vi "Connect.vi"(8 "error in (no error)":errorcluster, 11 "Red Pitaya in":refnum<class "Red Pitaya.lvclass">) -> (0 "error out":errorcluster, 3 "Red Pitaya out":refnum<class "Red Pitaya.lvclass">)   [LabVIEW 2015]
uses:
  Mag Lab Measure/Mag Lab Error Handler/Mag Lab Error Handler.lvclass
  Red Pitaya.lvclass
panel:
  out "Server  output":string
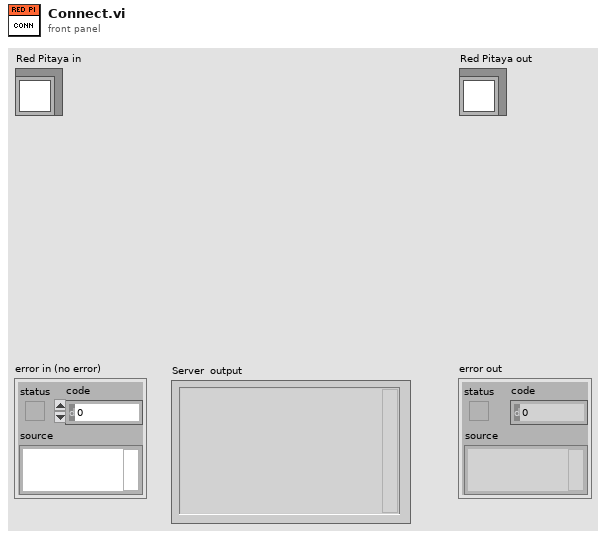
[diagram p1: front panel]
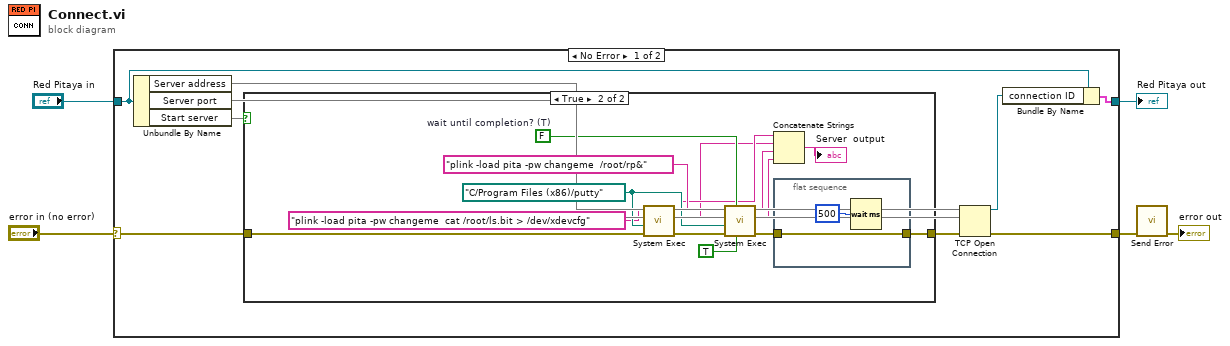
[diagram p0: block diagram]
diagram:
  n1 = case shown="No Error" "error in (no error)" {
    selector: "error in (no error)" -> [w7 w33]
    tunnel: [w11 w33] -> w4
    tunnel: [w13 w32] -> w2
    tunnel: "Red Pitaya in" -> [w14 w32]
    frame No Error {
      n2 = Unbundle By Name(w14) -> ("Server address"=w10, "Server port"=w9, "Start server"=w8)
      n3 = case shown="True" w8 {
        tunnel: [w15 w23] -> w6
        tunnel: w7 -> [w15 w21]
        frame False {
        }
        frame True {
          w22 = FALSE  # wait until completion? (T)
          w19 = path "C:/Program Files (x86)/putty" ("working directory")
          n4 = call <vilib>:"System Exec.vi"("error in (no error)"=w21, "working directory"=w19, "command line"="plink -load pita -pw changeme  cat /root/ls.bit > /dev/xdevcfg") -> ("error out"=w20:errorcluster, "standard error"=w16:string, "standard output"=w17:string)  [unwired: 5 in, 1 out]
          n5 = call <vilib>:"System Exec.vi"("run minimized? (F)"=TRUE, "wait until completion? (T)"=w22, "error in (no error)"=w20, "working directory"=w19, "command line"="plink -load pita -pw changeme  /root/rp&") -> ("error out"=w24:errorcluster, "standard error"=w26:string, "standard output"=w29:string)  [unwired: 3 in, 1 out]
          n6 = Concatenate Strings(w17, w16, w29, w26) -> (→"Server  output":string)
          n7 = flat-sequence {
            tunnel: w24 -> [w31]
            tunnel: [w31] -> w23
            frame #0 {
              n8 = Wait (ms)(milliseconds to wait=u32 500) -> ()  [unwired: 1 out]
            }
          }
        }
      }
      n9 = TCP Open Connection(address=w10, remote port or service name=w9, error in (no error)=w6) -> (connection ID=w12:refnum<k5>, error out=w11:errorcluster)  [unwired: 2 in]
      n10 = Bundle By Name(cluster=w14, "connection ID"=w12) -> (w13:cluster{})
    }
    frame Error {
    }
  }
  "Red Pitaya out" <- w2
  n11 = call "Send Error.vi"("error in (no error)"=w4) -> ("error out"=→"error out":errorcluster)  [unwired: 9 in, 1 out]
